vi "Pitot-static_to_Velocity.vi"(0 "Pressure Trans voltage":dbl[](array[numeric]) format="%.2f", 1 "Stat gauge Press mmH2O  (0)":dbl format="%.1f", 2 "Atmos Press mbar  (1000)":dbl=1000.0 format="%.1f", 3 "Temp  C  (20)":dbl=20.0 format="%.1f", 4 "Pressure Trans Calib const":dbl[](array[numeric]) format="%.6f") -> (5 "Velocity (m/s)":dbl[](array[numeric]) format="%.2f", 7 "Density Kg/m3":dbl format="%.2f")   [LabVIEW 2012]
doc: "this vi calculates the fluid velocity from the dynamic pressure measured with a pitot tube. Given a voltage array from the micro manometer and its calibration constants, it calculates the dynamic pressure, and knowing the temperature and absolute pressure of the fluid, calculates its velocity."
uses:
  Controls/Pressure_Units.ctl
panel:
  # "A              B"
  # "Instrument by PH. 18/2/94"
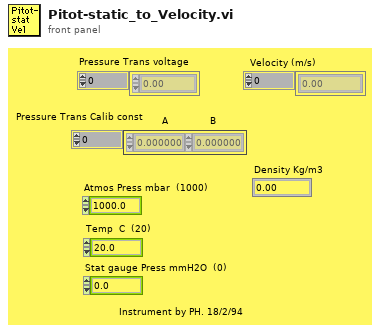
[diagram p1: front panel]
types:
  T1 = typedef "Pressure_Units.ctl" = enum16{"mmH2O", "mmHg", "Pa (N/m^2)", "mbar", "bar"}
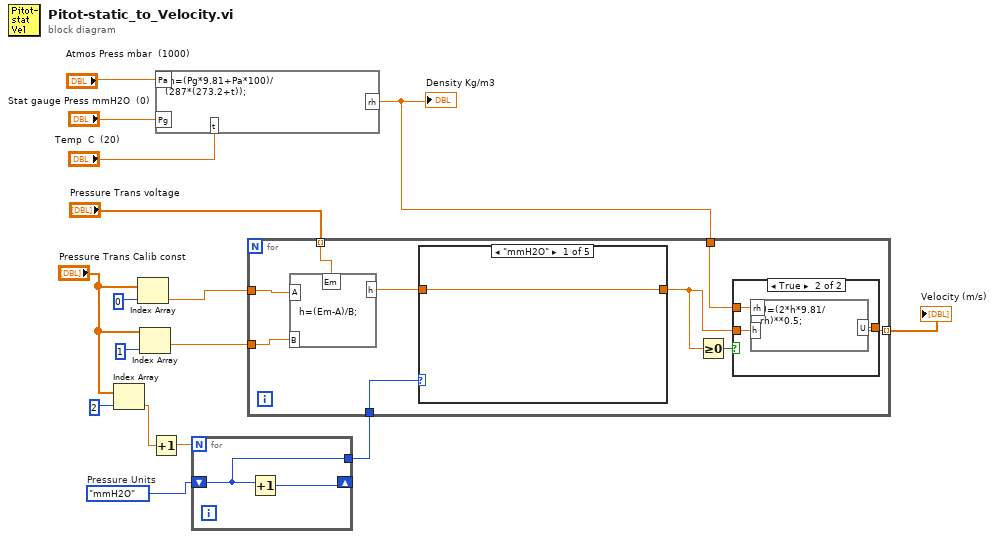
[diagram p0: block diagram]
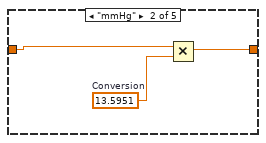
[diagram p2: hidden frame]
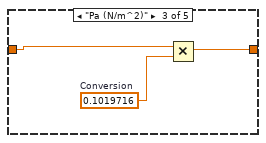
[diagram p3: hidden frame]
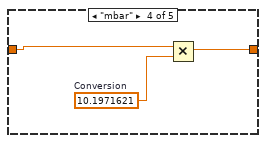
[diagram p4: hidden frame]
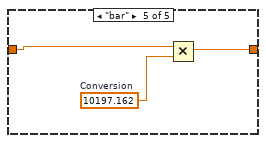
[diagram p5: hidden frame]
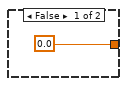
[diagram p6: hidden frame]
diagram:
  w4 = Pressure_Units."mmH2O"  # Pressure Units
  n1 = Index Array(array="Pressure Trans Calib const", index=2) -> (element=w3:dbl)
  n2 = Index Array(array="Pressure Trans Calib const", index=0) -> (element=w8:dbl)
  n3 = Index Array(array="Pressure Trans Calib const", index=1) -> (element=w7:dbl)
  n4 = Increment(x=w3) -> (x+1=w1:dbl)
  n5 = formula code="rh=(Pg*9.81+Pa*100)/\n(287*(273.2+t));"("t"="Temp  C  (20)", "Pg"="Stat gauge Press mmH2O  (0)", "Pa"="Atmos Press mbar  (1000)") -> ("rh"=w12:dbl)
  "Density Kg/m3" <- w12
  n6 = for {
    N: w1 -> [_]
    shift-right: [w18] -> _
    shift-left: w4 -> [w17]
    tunnel: [w17] -> w2
    n7 = Increment(x=w17) -> (x+1=w18:T1)
  }
  n8 = for {
    tunnel: [w23] -> w11 mode=indexing
    tunnel: w12 -> [w24]
    tunnel: "Pressure Trans voltage" -> [w25] mode=indexing
    tunnel: w7 -> [w26]
    tunnel: w8 -> [w27]
    tunnel: w2 -> [w21]
    n9 = formula code="h=(Em-A)/B;"("Em"=w25, "B"=w26, "A"=w27) -> ("h"=w20:dbl)
    n10 = case shown="\"mmH2O\"" w21 {
      tunnel: [w28 w30 w33 w36 w39] -> w19
      tunnel: w20 -> [w28 w31 w34 w37 w40]
      frame "mmH2O" {
      }
      frame "mmHg" {
        w29 = 13.5951  # Conversion
        n11 = Multiply(x=w31, y=w29) -> (x*y=w30:dbl)
      }
      frame "Pa (N/m^2)" {
        w32 = 0.1019716  # Conversion
        n12 = Multiply(x=w34, y=w32) -> (x*y=w33:dbl)
      }
      frame "mbar" {
        w35 = 10.1971621  # Conversion
        n13 = Multiply(x=w37, y=w35) -> (x*y=w36:dbl)
      }
      frame "bar" {
        w38 = 10197.162  # Conversion
        n14 = Multiply(x=w40, y=w38) -> (x*y=w39:dbl)
      }
    }
    n15 = Greater Or Equal To 0?(x=w19) -> (x >= 0?=w22:bool)
    n16 = case shown="True" w22 {
      tunnel: w24 -> [_ w44]
      tunnel: [0.0 w43] -> w23
      tunnel: w19 -> [_ w42]
      frame False {
      }
      frame True {
        n17 = formula code="U=(2*h*9.81/rh)**0.5;"("rh"=w44, "h"=w42) -> ("U"=w43:dbl)
      }
    }
  }
  "Velocity (m/s)" <- w11
